vi "Zoom Issue (LV2023Q3).vi"() -> ()   [LabVIEW 2023]
panel:
  in  "Directory Tree":string(tree)
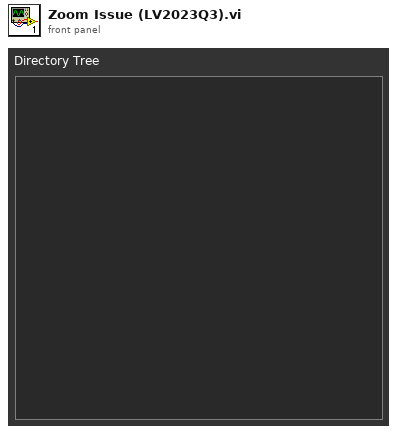
[diagram p1: front panel]
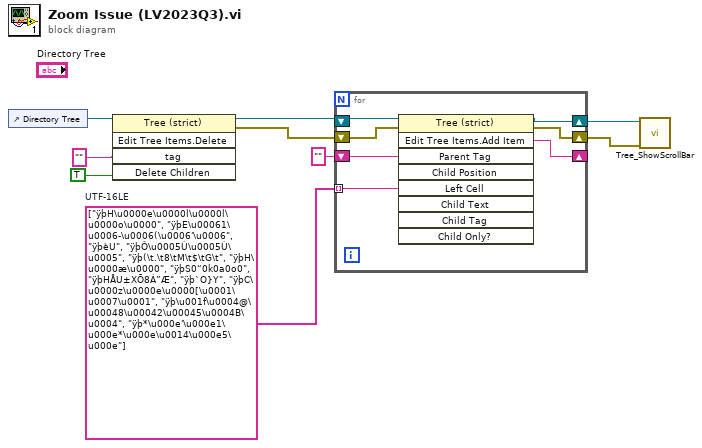
[diagram p0: block diagram]
diagram:
  w2 = string[] ["ÿþH\u0000e\u0000l\u0000l\u0000o\u0000", "ÿþE\u00061\u0006-\u0006(\u0006'\u0006", "ÿþèU", "ÿþÔ\u0005Ù\u0005Ù\u0005", "ÿþ(\t.\t8\tM\t$\tG\t", "ÿþH\u0000æ\u0000", "ÿþS0“0k0a0o0", "ÿþHÅU±XÕ8Á”Æ", "ÿþ`O}Y", "ÿþC\u0000z\u0000e\u0000[\u0001\u0007\u0001", "ÿþ\u001f\u0004@\u00048\u00042\u00045\u0004B\u0004", "ÿþ*\u000e'\u000e1\u000e*\u000e\u0014\u000e5\u000e"]  # UTF-16LE
  n1 = control-ref of="Directory Tree"() -> (w3:refnum<vi>)
  n2 = invoke class="Tree (strict)" method="Edit Tree Items.Delete"(reference=w3, "tag"="" ("Tag"), "Delete Children"=TRUE ("Delete Children?")) -> (reference out=w9:refnum<vi>, error out=w6:errorcluster)  [unwired: 2 in, 3 out]
  n3 = for {
    tunnel: w2 -> [w14] mode=indexing
    shift-right: [w13] -> w5
    shift-left: w9 -> [w16]
    shift-right: [w12] -> _
    shift-left: "" ("Edit Tree Items:Add Item") -> [w11]
    shift-right: [w10] -> w1
    shift-left: w6 -> [w15]
    n4 = invoke class="Tree (strict)" method="Edit Tree Items.Add Item"(reference=w16, error in=w15, "Parent Tag"=w11, "Left Cell"=w14) -> (reference out=w13:refnum<vi>, error out=w10:errorcluster, "Edit Tree Items:Add Item"=w12:string)  [unwired: 5 in, 6 out]
  }
  n5 = call <vilib>:"Tree_ShowScrollBar.vi"("error in (no error)"=w1, "Tree"=w5) -> ()  [unwired: 9 in, 1 out]
